vi "绘制判定框.vi"(7 "曲线引用":refnum<vi>, 8 "error in (no error)":errorcluster caption="错误输入（无错误）", 10 "判定框类型":enum16{"区间", "终点"}(ring), 11 "曲线判定条件":T1) -> (0 "error out":errorcluster caption="错误输出", 3 "判定框":cluster{"横坐标":dbl[], "纵坐标":dbl[]}[](array[cluster]))   [LabVIEW 2018]
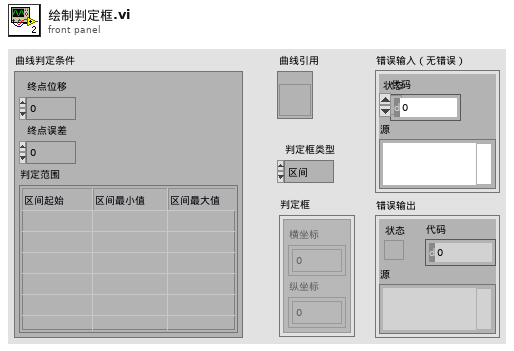
[diagram p1: front panel]
types:
  T1 = cluster{"终点位移":dbl, "终点误差":dbl, "判定范围":string[][]}
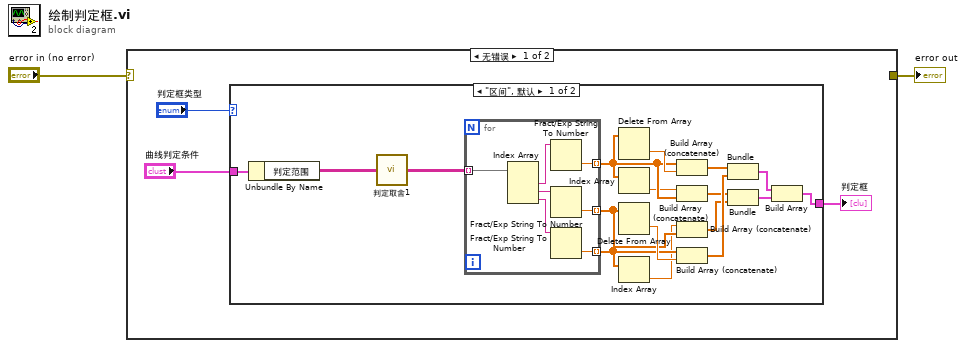
[diagram p0: block diagram]
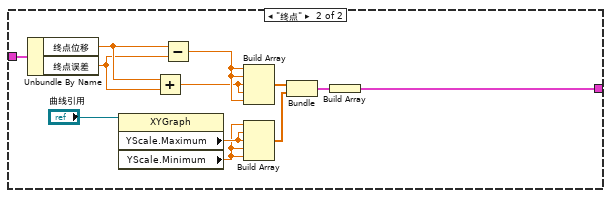
[diagram p2: hidden frame]
diagram:
  n1 = case shown="无错误" "error in (no error)" {
    selector: "error in (no error)" -> [_ w42]
    tunnel: [_ w42] -> w1
    frame No Error {
      n2 = case shown="\"区间\", 默认" "判定框类型" {
        tunnel: "曲线判定条件" -> [w22 w41]
        tunnel: [w13 w30] -> w3
        frame "区间", Default {
          n3 = Unbundle By Name(w22) -> ("判定范围"=w21:string[][])
          n4 = call "判定取舍1.vi"("输入表格"=w21) -> ("输出表格"=w20:string[][])
          n5 = for {
            tunnel: w20 -> [w29] mode=indexing
            tunnel: [w27] -> w9 mode=indexing
            tunnel: [w24] -> w10 mode=indexing
            tunnel: [w23] -> w7 mode=indexing
            n6 = Index Array(array=w29) -> (element #1=w28:string, element #2=w26:string, element #3=w25:string)  [unwired: 3 in]
            n7 = Fract/Exp String To Number(string=w28) -> (number=w27:dbl)  [unwired: 3 in, 1 out]
            n8 = Fract/Exp String To Number(string=w26) -> (number=w23:dbl)  [unwired: 3 in, 1 out]
            n9 = Fract/Exp String To Number(string=w25) -> (number=w24:dbl)  [unwired: 3 in, 1 out]
          }
          n10 = Delete From Array(array=w9) -> (deleted portion=w15:dbl)  [unwired: 2 in, 1 out]
          n11 = Index Array(array=w9) -> (element=w8:dbl)  [unwired: 1 in]
          n12 = Delete From Array(array=w7) -> (deleted portion=w14:dbl)  [unwired: 2 in, 1 out]
          n13 = Index Array(array=w10) -> (element=w6:dbl)  [unwired: 1 in]
          n14 = Build Array (concatenate)(w9, w15) -> (w19:dbl[])
          n15 = Build Array (concatenate)(w8, w9) -> (w16:dbl[])
          n16 = Build Array (concatenate)(w6, w7) -> (w17:dbl[])
          n17 = Build Array (concatenate)(w10, w14) -> (w18:dbl[])
          n18 = Bundle(w19, w18) -> (w12:cluster{dbl[], dbl[]})  [unwired: 1 in]
          n19 = Bundle(w16, w17) -> (w11:cluster{dbl[], dbl[]})  [unwired: 1 in]
          n20 = Build Array(w12, w11) -> (w13:cluster{dbl[], dbl[]}[])
        }
        frame "终点" {
          n21 = Unbundle By Name(w41) -> ("终点位移"=w40:dbl, "终点误差"=w39:dbl)
          n22 = property class="XYGraph"(reference="曲线引用") -> ("YScale.Maximum"=w34:dbl, "YScale.Minimum"=w33:dbl)  [unwired: 1 in, 2 out]
          n23 = Add(x=w40, y=w39) -> (x+y=w37:dbl)
          n24 = Subtract(x=w40, y=w39) -> (x-y=w38:dbl)
          n25 = Build Array(w38, w38, w37, w37, w38) -> (w36:dbl[])
          n26 = Build Array(w33, w34, w34, w33, w33) -> (w32:dbl[])
          n27 = Bundle(w36, w32) -> (w31:cluster{dbl[], dbl[]})  [unwired: 1 in]
          n28 = Build Array(w31) -> (w30:cluster{dbl[], dbl[]}[])
        }
      }
      "判定框" <- w3
    }
    frame Error {
    }
  }
  "error out" <- w1
